vi "LC-MISDK_GetSampleData.vi"() -> ()   [LabVIEW 2015]
uses:
  C:/Users/e09031/Documents/GMA/LC-160/Labview/Sample_LC-MISDK/LC-MISDK.dll
  LC-MISDK.dll
panel:
  in  "EXIT":bool
  out "Sample Data":string[][](table) caption="表"
  in  "GetSampleData":bool
  out "DataNum":dbl
  in  "ColorSpace":T1(ring)
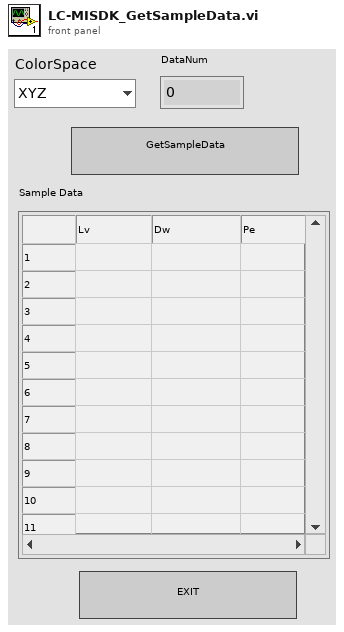
[diagram p1: front panel]
types:
  T1 = enum16{"XYZ", "Lvxy", "Lvudvd", "LvTcpDuv", "LvDwPe"}
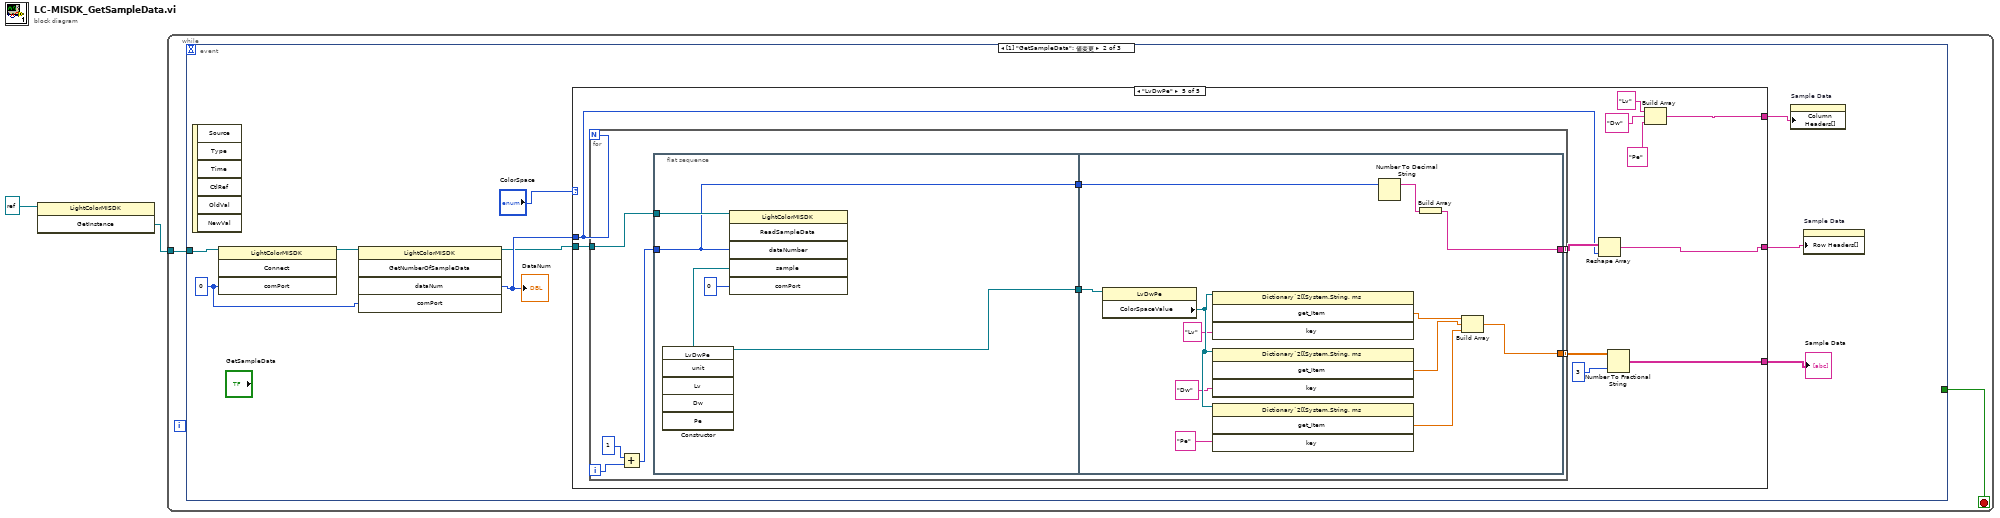
[diagram p0: block diagram]
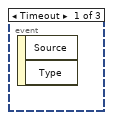
[diagram p2: hidden frame]
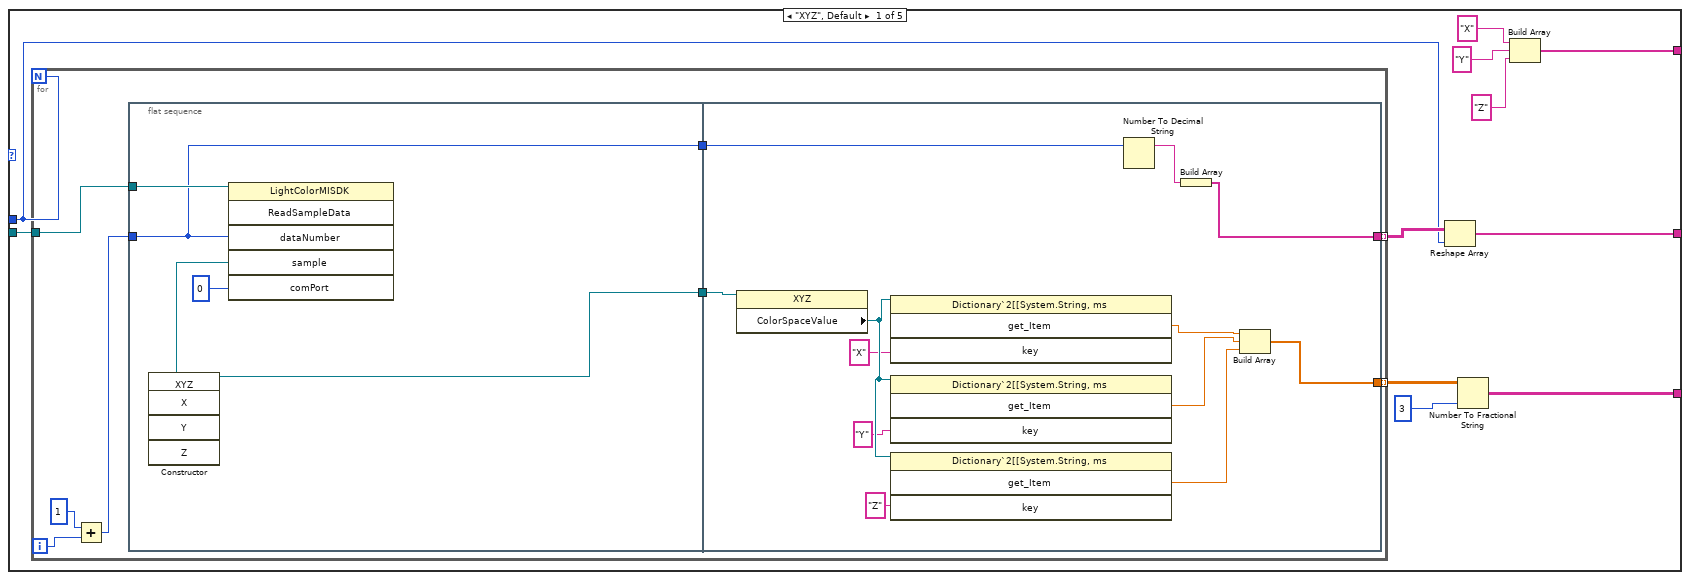
[diagram p3: hidden frame]
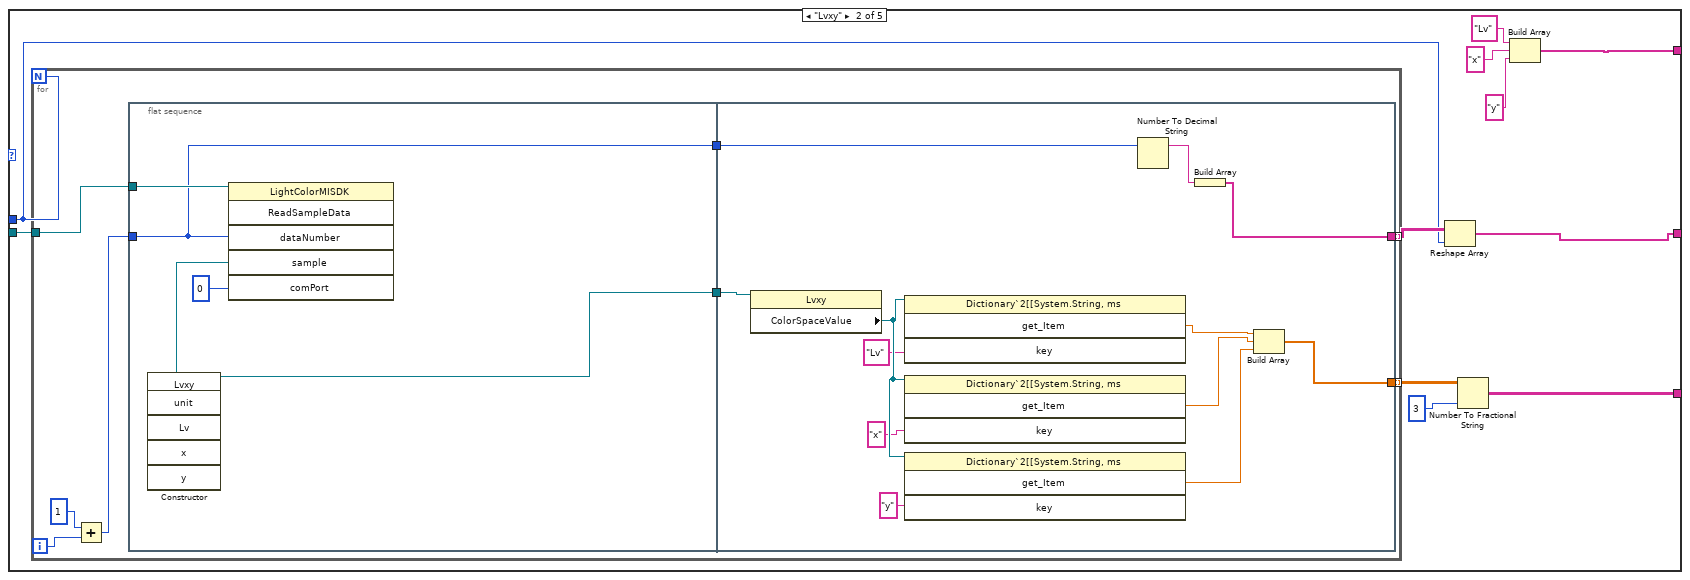
[diagram p4: hidden frame]
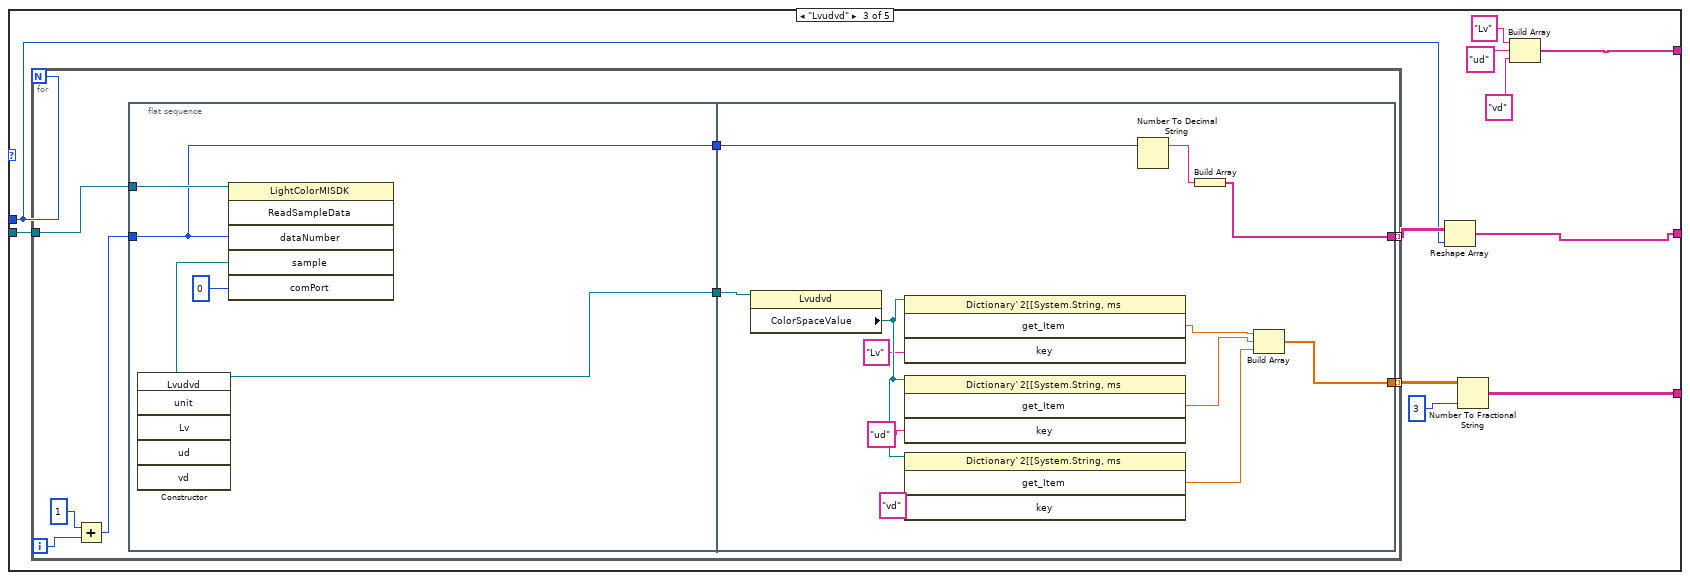
[diagram p5: hidden frame]
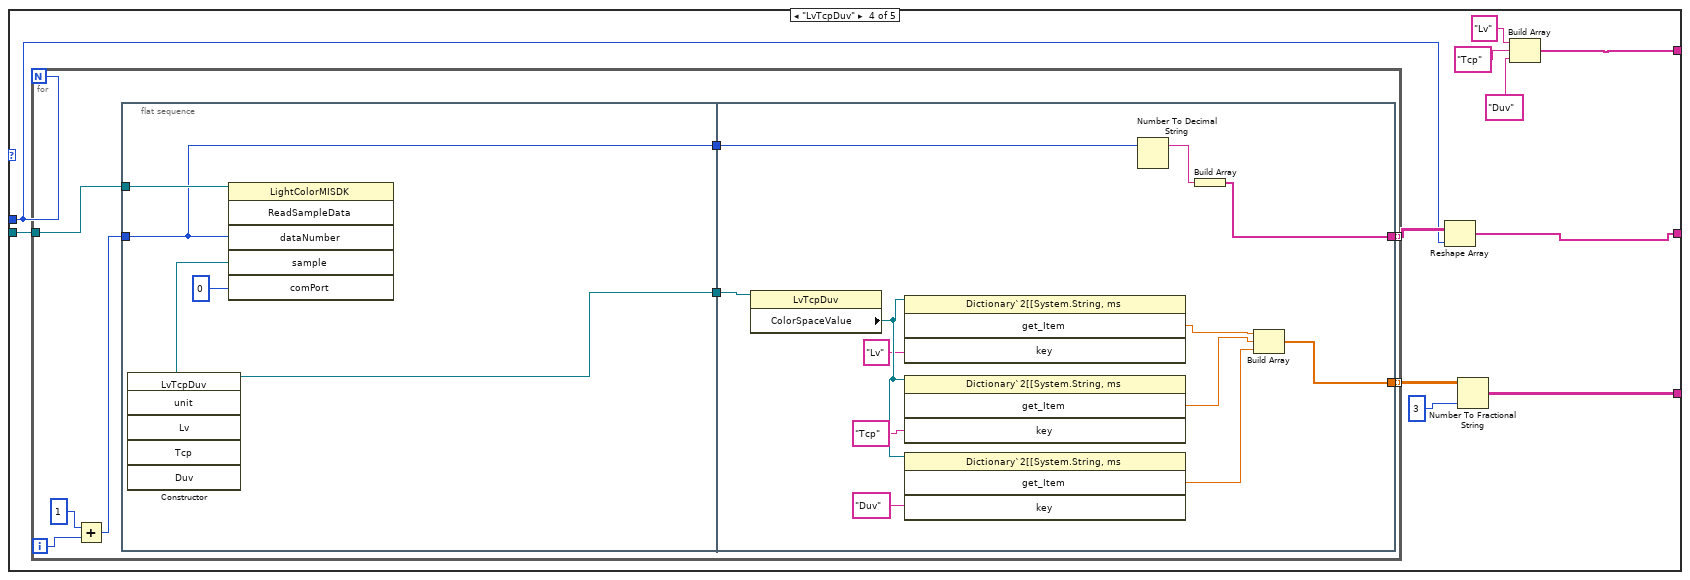
[diagram p6: hidden frame]
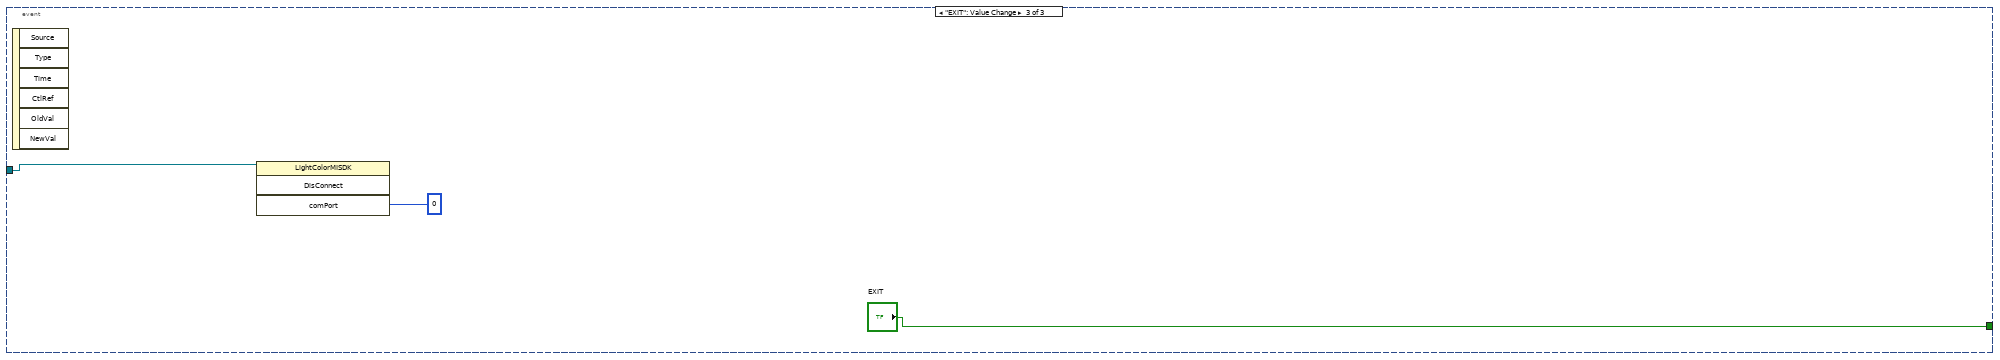
[diagram p7: hidden frame]
diagram:
  n1 = invoke on="インボークノード" class="LightColorMISDK" method="GetInstance"(reference=refnum<k24> refnum ("GetInstance")) -> ("GetInstance"=w1:refnum<k24>)  [unwired: 2 in, 2 out]
  n2 = while {
    tunnel: w1 -> [w4]
    stop <- w3 stop-if-true
    n3 = event shown="[1] \"GetSampleData\": 値変更" {
      selector: _ -> [_ _ _]
      dyn-events: _ -> [_ _ _]
      timeout: _ -> [_ _ _]
      tunnel: w4 -> [_ w13 w190]
      tunnel: [_ _ "EXIT"] -> w3
      event Timeout {
        n4 = event-data() -> ()  [unwired: 1 in, 2 out]
      }
      event "GetSampleData": Value Change {
        w11 = 0
        n5 = event-data() -> ()  [unwired: 1 in, 6 out]
        n6 = invoke on="インボークノード" class="LightColorMISDK" method="Connect"(reference=w13, "comPort"=w11) -> (reference out=w12:refnum<k24>)  [unwired: 2 in, 3 out]
        n7 = invoke on="インボークノード" class="LightColorMISDK" method="GetNumberOfSampleData"(reference=w12, "comPort"=w11) -> (reference out=w8:refnum<k24>, "dataNum"=w9:i32)  [unwired: 3 in, 3 out]
        "DataNum" <- w9
        n8 = case shown="\"LvDwPe\"" "ColorSpace" {
          tunnel: w9 -> [w17 w52 w87 w122 w157]
          tunnel: w8 -> [w24 w59 w94 w129 w164]
          tunnel: [w16 w51 w86 w121 w156] -> w7
          tunnel: [w15 w50 w85 w120 w155] -> w6
          tunnel: [w14 w49 w84 w119 w154] -> w5
          frame "XYZ", Default {
            n9 = for {
              N: w17 -> [_]
              tunnel: w24 -> [w32]
              tunnel: [w27] -> w22 mode=indexing
              tunnel: [w25] -> w18 mode=indexing
              i -> [w31]
              n10 = Add(x=1, y=w31) -> (x+y=w29:i32)
              n11 = flat-sequence {
                tunnel: w32 -> [w35]
                tunnel: w29 -> [w33]
                tunnel: [w34] -> w28
                tunnel: [w33] -> w26
                tunnel: w28 -> [w41]
                tunnel: [w40] -> w27
                tunnel: w26 -> [w39]
                tunnel: [w37] -> w25
                frame #0 {
                  n12 = constructor class="XYZ"() -> (reference out=w34:refnum<k24>)  [unwired: 6 in, 5 out]
                  n13 = invoke on="インボークノード" class="LightColorMISDK" method="ReadSampleData"(reference=w35, "dataNumber"=w33, "sample"=w34, "comPort"=0) -> ()  [unwired: 2 in, 6 out]
                }
                frame #1 {
                  n14 = property on="プロパティノード" class="XYZ"(reference=w41) -> ("ColorSpaceValue"=w48:refnum<k24>)  [unwired: 1 in, 2 out]
                  n15 = invoke class="Dictionary`2[[System.String, ms" method="get_Item"(reference=w48, "key"="X") -> ("get_Item"=w42:dbl)  [unwired: 2 in, 3 out]
                  n16 = invoke class="Dictionary`2[[System.String, ms" method="get_Item"(reference=w48, "key"="Y") -> ("get_Item"=w44:dbl)  [unwired: 2 in, 3 out]
                  n17 = invoke class="Dictionary`2[[System.String, ms" method="get_Item"(reference=w48, "key"="Z") -> ("get_Item"=w43:dbl)  [unwired: 2 in, 3 out]
                  n18 = Number To Decimal String(number=w39) -> (decimal integer string=w38:string)  [unwired: 1 in]
                  n19 = Build Array(w38) -> (w37:string[])
                  n20 = Build Array(w42, w44, w43) -> (w40:dbl[])
                }
              }
            }
            n21 = Reshape Array(w18, w17) -> (w14:string[])
            n22 = Number To Fractional String(number=w22, precision (6)=3) -> (F-format string=w16:string[][])  [unwired: 2 in]
            n23 = Build Array("X", "Y", "Z") -> (w15:string[])
          }
          frame "Lvxy" {
            n24 = for {
              N: w52 -> [_]
              tunnel: w59 -> [w67]
              tunnel: [w62] -> w57 mode=indexing
              tunnel: [w60] -> w53 mode=indexing
              i -> [w66]
              n25 = Add(x=1, y=w66) -> (x+y=w64:i32)
              n26 = flat-sequence {
                tunnel: w67 -> [w70]
                tunnel: w64 -> [w68]
                tunnel: [w69] -> w63
                tunnel: [w68] -> w61
                tunnel: w63 -> [w76]
                tunnel: [w75] -> w62
                tunnel: w61 -> [w74]
                tunnel: [w72] -> w60
                frame #0 {
                  n27 = constructor class="Lvxy"() -> (reference out=w69:refnum<k24>)  [unwired: 7 in, 6 out]
                  n28 = invoke on="インボークノード" class="LightColorMISDK" method="ReadSampleData"(reference=w70, "dataNumber"=w68, "sample"=w69, "comPort"=0) -> ()  [unwired: 2 in, 6 out]
                }
                frame #1 {
                  n29 = property on="プロパティノード" class="Lvxy"(reference=w76) -> ("ColorSpaceValue"=w83:refnum<k24>)  [unwired: 1 in, 2 out]
                  n30 = invoke class="Dictionary`2[[System.String, ms" method="get_Item"(reference=w83, "key"="Lv") -> ("get_Item"=w77:dbl)  [unwired: 2 in, 3 out]
                  n31 = invoke class="Dictionary`2[[System.String, ms" method="get_Item"(reference=w83, "key"="x") -> ("get_Item"=w79:dbl)  [unwired: 2 in, 3 out]
                  n32 = invoke class="Dictionary`2[[System.String, ms" method="get_Item"(reference=w83, "key"="y") -> ("get_Item"=w78:dbl)  [unwired: 2 in, 3 out]
                  n33 = Number To Decimal String(number=w74) -> (decimal integer string=w73:string)  [unwired: 1 in]
                  n34 = Build Array(w73) -> (w72:string[])
                  n35 = Build Array(w77, w79, w78) -> (w75:dbl[])
                }
              }
            }
            n36 = Reshape Array(w53, w52) -> (w49:string[])
            n37 = Number To Fractional String(number=w57, precision (6)=3) -> (F-format string=w51:string[][])  [unwired: 2 in]
            n38 = Build Array("Lv", "x", "y") -> (w50:string[])
          }
          frame "Lvudvd" {
            n39 = for {
              N: w87 -> [_]
              tunnel: w94 -> [w102]
              tunnel: [w97] -> w92 mode=indexing
              tunnel: [w95] -> w88 mode=indexing
              i -> [w101]
              n40 = Add(x=1, y=w101) -> (x+y=w99:i32)
              n41 = flat-sequence {
                tunnel: w102 -> [w105]
                tunnel: w99 -> [w103]
                tunnel: [w104] -> w98
                tunnel: [w103] -> w96
                tunnel: w98 -> [w111]
                tunnel: [w110] -> w97
                tunnel: w96 -> [w109]
                tunnel: [w107] -> w95
                frame #0 {
                  n42 = constructor class="Lvudvd"() -> (reference out=w104:refnum<k24>)  [unwired: 7 in, 6 out]
                  n43 = invoke on="インボークノード" class="LightColorMISDK" method="ReadSampleData"(reference=w105, "dataNumber"=w103, "sample"=w104, "comPort"=0) -> ()  [unwired: 2 in, 6 out]
                }
                frame #1 {
                  n44 = property on="プロパティノード" class="Lvudvd"(reference=w111) -> ("ColorSpaceValue"=w118:refnum<k24>)  [unwired: 1 in, 2 out]
                  n45 = invoke class="Dictionary`2[[System.String, ms" method="get_Item"(reference=w118, "key"="Lv") -> ("get_Item"=w112:dbl)  [unwired: 2 in, 3 out]
                  n46 = invoke class="Dictionary`2[[System.String, ms" method="get_Item"(reference=w118, "key"="ud") -> ("get_Item"=w114:dbl)  [unwired: 2 in, 3 out]
                  n47 = invoke class="Dictionary`2[[System.String, ms" method="get_Item"(reference=w118, "key"="vd") -> ("get_Item"=w113:dbl)  [unwired: 2 in, 3 out]
                  n48 = Number To Decimal String(number=w109) -> (decimal integer string=w108:string)  [unwired: 1 in]
                  n49 = Build Array(w108) -> (w107:string[])
                  n50 = Build Array(w112, w114, w113) -> (w110:dbl[])
                }
              }
            }
            n51 = Reshape Array(w88, w87) -> (w84:string[])
            n52 = Number To Fractional String(number=w92, precision (6)=3) -> (F-format string=w86:string[][])  [unwired: 2 in]
            n53 = Build Array("Lv", "ud", "vd") -> (w85:string[])
          }
          frame "LvTcpDuv" {
            n54 = for {
              N: w122 -> [_]
              tunnel: w129 -> [w137]
              tunnel: [w132] -> w127 mode=indexing
              tunnel: [w130] -> w123 mode=indexing
              i -> [w136]
              n55 = Add(x=1, y=w136) -> (x+y=w134:i32)
              n56 = flat-sequence {
                tunnel: w137 -> [w140]
                tunnel: w134 -> [w138]
                tunnel: [w139] -> w133
                tunnel: [w138] -> w131
                tunnel: w133 -> [w146]
                tunnel: [w145] -> w132
                tunnel: w131 -> [w144]
                tunnel: [w142] -> w130
                frame #0 {
                  n57 = constructor class="LvTcpDuv"() -> (reference out=w139:refnum<k24>)  [unwired: 7 in, 6 out]
                  n58 = invoke on="インボークノード" class="LightColorMISDK" method="ReadSampleData"(reference=w140, "dataNumber"=w138, "sample"=w139, "comPort"=0) -> ()  [unwired: 2 in, 6 out]
                }
                frame #1 {
                  n59 = property on="プロパティノード" class="LvTcpDuv"(reference=w146) -> ("ColorSpaceValue"=w153:refnum<k24>)  [unwired: 1 in, 2 out]
                  n60 = invoke class="Dictionary`2[[System.String, ms" method="get_Item"(reference=w153, "key"="Lv") -> ("get_Item"=w147:dbl)  [unwired: 2 in, 3 out]
                  n61 = invoke class="Dictionary`2[[System.String, ms" method="get_Item"(reference=w153, "key"="Tcp") -> ("get_Item"=w149:dbl)  [unwired: 2 in, 3 out]
                  n62 = invoke class="Dictionary`2[[System.String, ms" method="get_Item"(reference=w153, "key"="Duv") -> ("get_Item"=w148:dbl)  [unwired: 2 in, 3 out]
                  n63 = Number To Decimal String(number=w144) -> (decimal integer string=w143:string)  [unwired: 1 in]
                  n64 = Build Array(w143) -> (w142:string[])
                  n65 = Build Array(w147, w149, w148) -> (w145:dbl[])
                }
              }
            }
            n66 = Reshape Array(w123, w122) -> (w119:string[])
            n67 = Number To Fractional String(number=w127, precision (6)=3) -> (F-format string=w121:string[][])  [unwired: 2 in]
            n68 = Build Array("Lv", "Tcp", "Duv") -> (w120:string[])
          }
          frame "LvDwPe" {
            n69 = for {
              N: w157 -> [_]
              tunnel: w164 -> [w172]
              tunnel: [w167] -> w162 mode=indexing
              tunnel: [w165] -> w158 mode=indexing
              i -> [w171]
              n70 = Add(x=1, y=w171) -> (x+y=w169:i32)
              n71 = flat-sequence {
                tunnel: w172 -> [w175]
                tunnel: w169 -> [w173]
                tunnel: [w174] -> w168
                tunnel: [w173] -> w166
                tunnel: w168 -> [w181]
                tunnel: [w180] -> w167
                tunnel: w166 -> [w179]
                tunnel: [w177] -> w165
                frame #0 {
                  n72 = constructor class="LvDwPe"() -> (reference out=w174:refnum<k24>)  [unwired: 7 in, 6 out]
                  n73 = invoke on="インボークノード" class="LightColorMISDK" method="ReadSampleData"(reference=w175, "dataNumber"=w173, "sample"=w174, "comPort"=0) -> ()  [unwired: 2 in, 6 out]
                }
                frame #1 {
                  n74 = property on="プロパティノード" class="LvDwPe"(reference=w181) -> ("ColorSpaceValue"=w188:refnum<k24>)  [unwired: 1 in, 2 out]
                  n75 = invoke class="Dictionary`2[[System.String, ms" method="get_Item"(reference=w188, "key"="Lv") -> ("get_Item"=w182:dbl)  [unwired: 2 in, 3 out]
                  n76 = invoke class="Dictionary`2[[System.String, ms" method="get_Item"(reference=w188, "key"="Dw") -> ("get_Item"=w184:dbl)  [unwired: 2 in, 3 out]
                  n77 = invoke class="Dictionary`2[[System.String, ms" method="get_Item"(reference=w188, "key"="Pe") -> ("get_Item"=w183:dbl)  [unwired: 2 in, 3 out]
                  n78 = Number To Decimal String(number=w179) -> (decimal integer string=w178:string)  [unwired: 1 in]
                  n79 = Build Array(w178) -> (w177:string[])
                  n80 = Build Array(w182, w184, w183) -> (w180:dbl[])
                }
              }
            }
            n81 = Reshape Array(w158, w157) -> (w154:string[])
            n82 = Number To Fractional String(number=w162, precision (6)=3) -> (F-format string=w156:string[][])  [unwired: 2 in]
            n83 = Build Array("Lv", "Dw", "Pe") -> (w155:string[])
          }
        }
        "Sample Data" <- w7
        n84 = property on="Sample Data" class="Tbl （指定）"("Column Headers[]"=w6) -> ()  [unwired: 2 in, 2 out]
        n85 = property on="Sample Data" class="Tbl （指定）"("Row Headers[]"=w5) -> ()  [unwired: 2 in, 2 out]
      }
      event "EXIT": Value Change {
        n86 = event-data() -> ()  [unwired: 1 in, 6 out]
        n87 = invoke on="インボークノード" class="LightColorMISDK" method="DisConnect"(reference=w190, "comPort"=0) -> ()  [unwired: 2 in, 4 out]
      }
    }
  }
